vi "常规五参数状态告警区.vi"(11 "数组":u16[](array[numeric]) format="%04xH") -> (3 "状态告警区":T1)   [LabVIEW 2016, in "斯坦道仪器.lvlib"]
panel:
  # "共占用16 WORD"
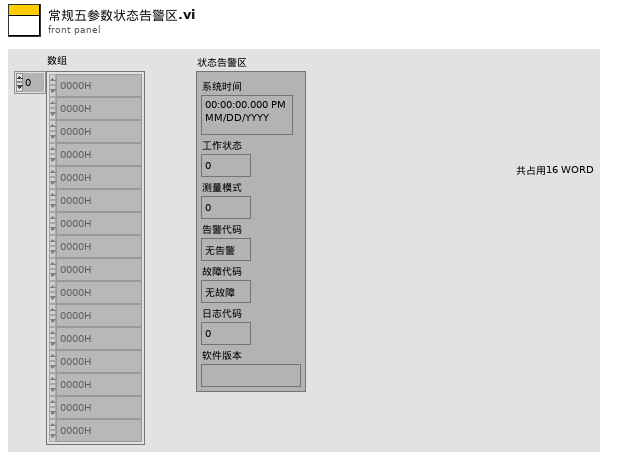
[diagram p1: front panel]
types:
  T1 = cluster{"系统时间":timestamp, "工作状态":u16, "测量模式":u16, "告警代码":enum16{"无告警", "缺试剂告警", "缺水样告警", "缺蒸馏水告警", "缺标液告警", "仪表漏液告警", "标定异常告警", "超量程告警", "加热异常", "低试剂预警", "超上限告警", "超下限告警", "仪表内部其他异常", "滴定异常告警", "电极异常告警", "量程切换告警", "参数设置告警", "PH电极电位异常", "电导率电极异常", "浊度光度异常", "溶解氧电极异常", "溶解氧光强异常", "温度异常告警", "PH异常告警", "溶解氧异常告警", "电导率异常告警", "浊度异常告警", "叶绿素异常告警", "藻密度异常告警", "蓝绿藻异常告警", "ORP异常告警", "氨氮异常告警", "清洁刷异常告警", "SD卡异常告警", "蓝牙异常告警", "Wifi异常告警", "流程异常告警"}, "故障代码":enum16{"无故障", "电机故障", "温度故障", "通讯故障", "滴定故障"}, "日志代码":u16, "软件版本":string}
  T2 = cluster{"time stamp":timestamp, "WORD":u16, "WORD":u16, "WORD":u16, "WORD":u16, "WORD":u16, "string":string}
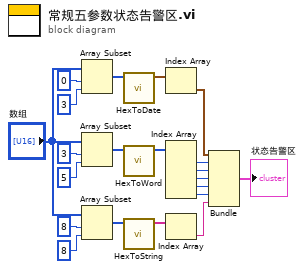
[diagram p0: block diagram]
diagram:
  n1 = Array Subset(array="数组", index=0 ("索引"), length=3 ("长度")) -> (w19:u16[])
  n2 = Array Subset(array="数组", index=3 ("索引"), length=5 ("长度")) -> (w14:u16[])
  n3 = Array Subset(array="数组", index=8 ("索引"), length=8 ("长度")) -> (w5:u16[])
  n4 = call "HexToDate.vi"("数组"=w19) -> ("DATE"=w16:timestamp[])  [unwired: 10 in]
  n5 = call "HexToWord.vi"("数组"=w14) -> ("WORD"=w13:u16[])  [unwired: 10 in]
  n6 = call "HexToString.vi"("数组"=w5) -> ("STRING"=w2:string[])  [unwired: 10 in]
  n7 = Index Array(array=w16) -> (element=w15:timestamp)  [unwired: 1 in]
  n8 = Index Array(array=w13) -> (element #1=w12:u16, element #2=w11:u16, element #3=w10:u16, element #4=w9:u16, element #5=w8:u16)  [unwired: 5 in]
  n9 = Index Array(array=w2) -> (element=w1:string)  [unwired: 1 in]
  n10 = Bundle("time stamp"=w15, "WORD"=w12, "WORD"=w11, "WORD"=w10, "WORD"=w9, "WORD"=w8, "string"=w1) -> (→"状态告警区":T2)  [unwired: 1 in]
